vi "MT Display 3DEye.vi"(0 "waveform":T2={"t0"=0.0, "dt"=1.0, "Y"=[]} {"Y" format="%.3f"; "dt" format="%^.2e"; "t0" format="%.4f"}, 1 "3D curve":refnum<k7>, 2 "clear graph":bool, 3 "optional settings":T1={"segment timing (ms)"=100, "occurrence refnum for abort"=refnum}, 5 "symbol rate (Hz)":dbl=1.0 format="%.2f", 7 "eye length (symbol periods)":i32=1, 9 "color":u32(colorbox)=6618880, 11 "error in (no error)":errorcluster, 12 "autoscale":bool, 13 "display size (segments)":i32=100) -> (15 "error out":errorcluster)   [LabVIEW 2020, in "niDMT.lvlib"]
doc: "Divides an input complex-valued waveform into segments and displays those segments as overlapping plots on a 3D graph. The VI determines the segment length based on the <B>symbol rate</B> and <B>eye length</B> parameters."
uses:
  <vilib>/addons/Modulation/niDMT.lvlib
  <vilib>/addons/Modulation/Analog/controls/Complex Data Waveform.ctl
  <vilib>/addons/Modulation/Digital/General/subVIs/mod_Segment Array(complex).vi
  <vilib>/Platform/NI_3dgraph.lvlib
  <vilib>/addons/Modulation/niAMT.lvlib
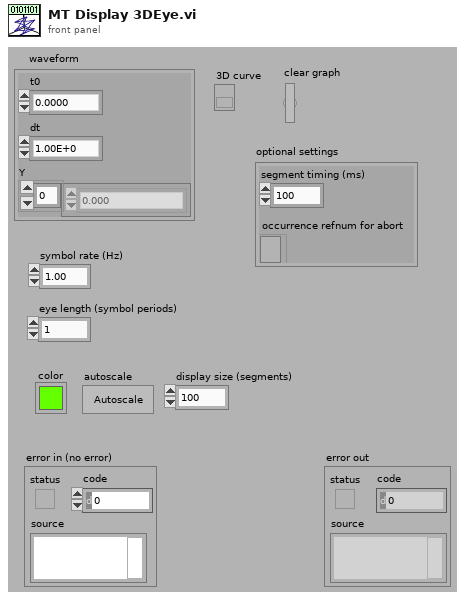
[diagram p1: front panel]
types:
  T1 = cluster{"segment timing (ms)":u32, "occurrence refnum for abort":refnum<k4>}
  T2 = typedef "niAMT.lvlib/Complex Data Waveform.ctl" = cluster{"t0":dbl, "dt":dbl, "Y":cdb[]}
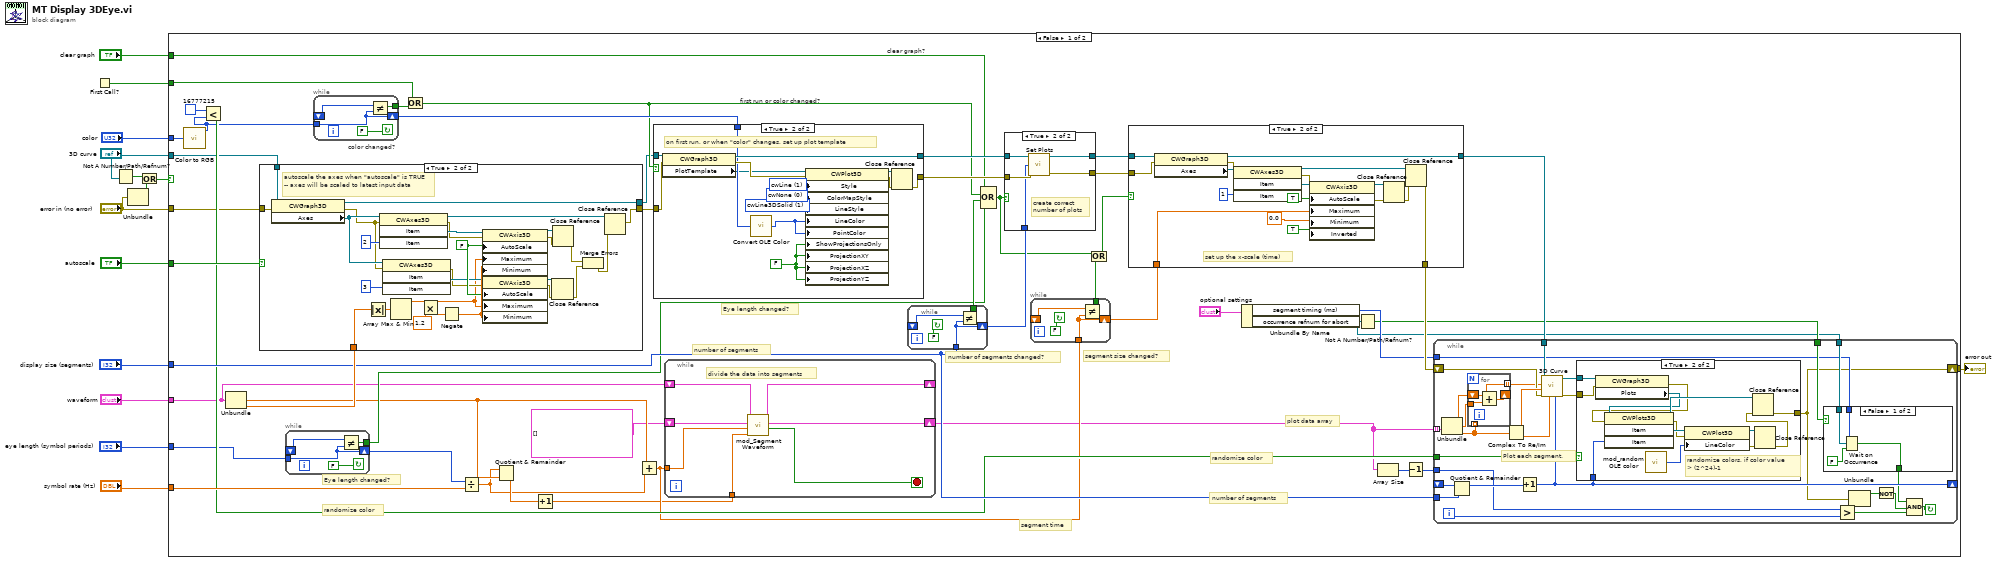
[diagram p0: block diagram]
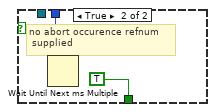
[diagram p2: hidden frame]
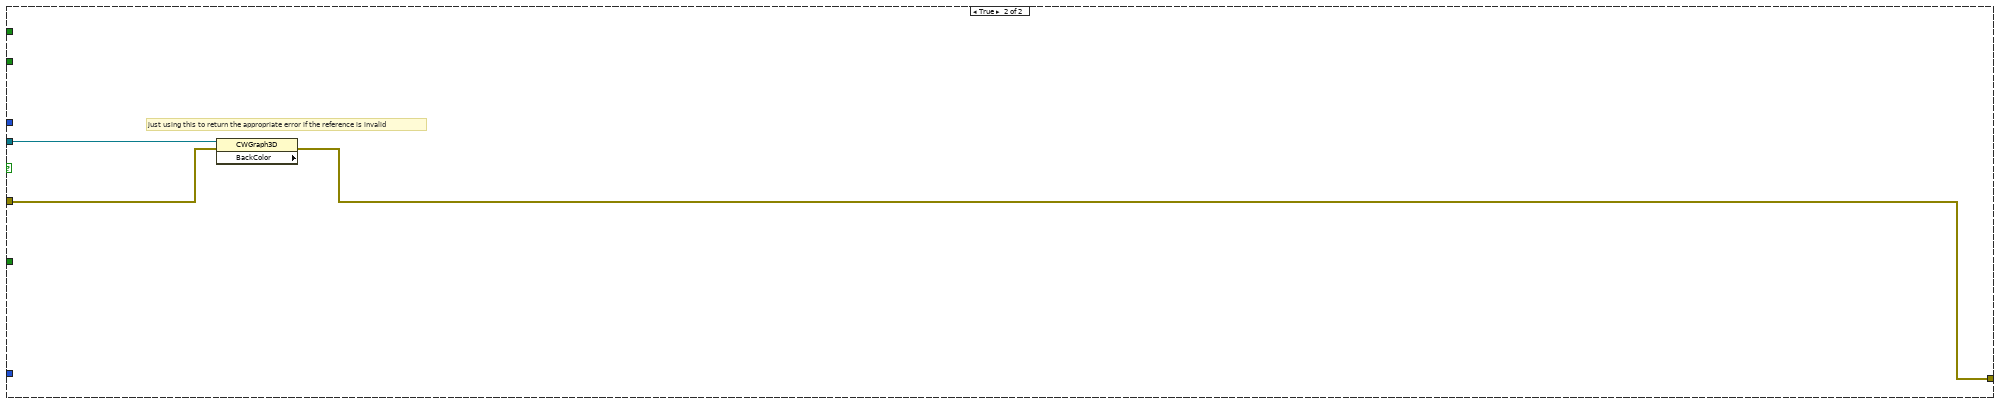
[diagram p8: hidden frame]
diagram:
  n1 = First Call?() -> (First Call?: T/F=w11:bool)
  n2 = Not A Number/Path/Refnum?(number/path/refnum="3D curve") -> (NaN/Path/Refnum?=w2:bool)
  n3 = Unbundle("error in (no error)") -> ("status"=w3:bool)  [unwired: 2 out]
  n4 = Or(x=w2, y=w3) -> (x .or. y?=w1:bool)
  n5 = case shown="False" w1 {
    tunnel: [w59 w206] -> w14
    tunnel: "symbol rate (Hz)" -> [w57 _]
    tunnel: "autoscale" -> [w56 _]
    tunnel: "3D curve" -> [w20 w208]
    tunnel: w11 -> [w51 _]
    tunnel: "display size (segments)" -> [w49 _]
    tunnel: "clear graph" -> [w48 _]
    tunnel: "eye length (symbol periods)" -> [w45 _]
    tunnel: "color" -> [w32 _]
    tunnel: "waveform" -> [w31 _]
    tunnel: "error in (no error)" -> [w26 w207]
    frame False {
      # "plot data array"
      # "number of segments"
      # "randomize color"
      # "segment time"
      # "clear graph?"
      # "first run or color changed?"
      # "Eye length changed?"
      # "number of segments"
      # "randomize color"
      # "segment size changed?"
      # "Eye length changed?"
      # "number of segments changed?"
      # "color changed?"
      n6 = call <vilib>:"Color to RGB.vi"("Color"=w32) -> ("Resolved Color"=w33:u32)  [unwired: 3 out]
      n7 = Less?(x=u32 16777215, y=w33) -> (x < y?=w46:bool)
      n8 = Unbundle(w31) -> ("dt"=w40:dbl, "Y"=w61:cdb[])  [unwired: 1 out]
      n9 = case shown="True" w56 {
        tunnel: w61 -> [_ w198]
        tunnel: w20 -> [w170 w188]
        tunnel: w26 -> [w171 w187]
        tunnel: [w171 w176] -> w27
        tunnel: [w170 w172] -> w19
        frame False {
        }
        frame True {
          w194 = FALSE ("AutoScale")
          # "autoscale the axes when \"autoscale\" is TRUE -- axes will be scaled to latest input data"
          n10 = property class="CWGraph3D"(reference=w188, error in=w187) -> (reference out=w172:refnum<k7>, error out=w185:errorcluster, "Axes"=w186:refnum<k7>)
          n11 = Absolute Value(x=w198) -> (abs(x)=w189:dbl[])
          n12 = invoke class="CWAxes3D" method="Item"(reference=w186, error in=w185, "Item"=2) -> (reference out=w178:refnum<k7>, error out=w184:errorcluster, "Item"=w192:refnum<k7>)  [unwired: 1 in, 1 out]
          n13 = invoke class="CWAxes3D" method="Item"(reference=w186, error in=w185, "Item"=3) -> (error out=w182:errorcluster, "Item"=w193:refnum<k7>)  [unwired: 1 in, 2 out]
          n14 = Array Max & Min(array=w189) -> (max value=w175:dbl)  [unwired: 3 out]
          n15 = Multiply(x=w175, y=1.2) -> (x*y=w174:dbl)
          n16 = Negate(x=w174) -> (-x=w195:dbl)
          n17 = property class="CWAxis3D"(reference=w192, error in=w184, "AutoScale"=w194, "Maximum"=w174, "Minimum"=w195) -> (reference out=w196:refnum<k7>, error out=w183:errorcluster)
          n18 = property class="CWAxis3D"(reference=w193, error in=w182, "AutoScale"=w194, "Maximum"=w174, "Minimum"=w195) -> (reference out=w197:refnum<k7>, error out=w181:errorcluster)
          n19 = Close Reference(reference=w197, error in (no error)=w181) -> (error out=w179:errorcluster)
          n20 = Close Reference(reference=w196, error in (no error)=w183) -> (error out=w180:errorcluster)
          n21 = Merge Errors(w180, w179) -> (w177:errorcluster)
          n22 = Close Reference(reference=w178, error in (no error)=w177) -> (error out=w176:errorcluster)
        }
      }
      n23 = while {
        shift-right: [w137] -> w44
        shift-left: _ -> [w138]
        tunnel: w45 -> [w137]
        tunnel: [w136] -> w43
        stop <- FALSE continue-if-true
        n24 = Not Equal?(x=w138, y=w137) -> (x != y?=w136:bool)
      }
      n25 = while {
        shift-right: [w141] -> w53
        shift-left: _ -> [w142]
        tunnel: w33 -> [w141]
        tunnel: [w140] -> w52
        stop <- FALSE continue-if-true
        n26 = Not Equal?(x=w142, y=w141) -> (x != y?=w140:bool)
      }
      n27 = Or(x=w51, y=w52) -> (x .or. y?=w50:bool)
      n28 = Divide(x=w44, y=w57) -> (x/y=w28:dbl)
      n29 = Quotient & Remainder(x=w28, y=w40) -> (floor(x/y)=w42:dbl)  [unwired: 1 out]
      n30 = Increment(x=w42) -> (x+1=w30:dbl)
      n31 = Add(x=w40, y=w28) -> (x+y=w41:dbl)
      n32 = case shown="True" w50 {
        tunnel: [w143 w145] -> w60
        tunnel: [w144 w158] -> w58
        tunnel: w53 -> [_ w154]
        tunnel: w19 -> [w144 w149]
        tunnel: w27 -> [w143 w148]
        frame False {
        }
        frame True {
          w151 = 1 items=["cwLine"=1, "cwPoint"=2, "cwLinePoint"=3, "cwHiddenLine"=4, "cwSurface"=5, "cwSurfaceLine"=6, "cwSurfaceNormal"=7, "cwContourLine"=8, "cwSurfaceContour"=9] ("Style")
          w152 = 0 items=["cwNone", "cwShaded", "cwColorSpectrum", "cwGrayScale", "cwCustom"] ("ColorMapStyle")
          w153 = 1 items=["cwLine3DNone"=0, "cwLine3DSolid"=1, "cwLine3DDash"=4, "cwLine3DDot"=5, "cwLine3DDashDot"=6] ("LineStyle")
          w157 = FALSE ("ShowProjectionsOnly")
          # "on first run, or when \"color\" changes, set up plot template"
          n33 = property class="CWGraph3D"(reference=w149, error in=w148) -> (reference out=w158:refnum<k7>, error out=w156:errorcluster, "PlotTemplate"=w150:refnum<k7>)
          n34 = call <vilib>:"Convert OLE Color.vi"("color in"=w154) -> ("color out"=w147:u32)
          n35 = property class="CWPlot3D"(reference=w150, error in=w156, "Style"=w151, "ColorMapStyle"=w152, "LineStyle"=w153, "LineColor"=w147, "PointColor"=w147, "ShowProjectionsOnly"=w157, "ProjectionXY"=w157, "ProjectionXZ"=w157, "ProjectionYZ"=w157) -> (reference out=w155:refnum<k7>, error out=w146:errorcluster)
          n36 = Close Reference(reference=w155, error in (no error)=w146) -> (error out=w145:errorcluster)
        }
      }
      n37 = while {
        tunnel: w41 -> [w201]
        shift-right: [w202] -> w24
        shift-left: cluster{dbl, "dt":dbl, cdb[]}[] [] -> [w203]
        shift-right: [w204] -> _
        shift-left: w31 -> [w205]
        tunnel: w30 -> [w200]
        stop <- w199 stop-if-true
        # "divide the data into segments"
        n38 = call-poly <vilib>:"mod_Segment Waveform.vi"("min samples per segment"=w200, "segment time"=w201, "graphs in"=w203, "waveform"=w205) -> ("done?"=w199:bool, "graphs out"=w202:cluster{dbl, "dt":dbl, cdb[]}[], "waveform out"=w204:cluster{"t0":dbl, "dt":dbl, "Y":cdb[]})  [unwired: 5 out]
      }
      n39 = while {
        shift-right: [w168] -> w55
        shift-left: _ -> [w169]
        tunnel: w49 -> [w168]
        tunnel: [w167] -> w54
        stop <- FALSE continue-if-true
        n40 = Not Equal?(x=w169, y=w168) -> (x != y?=w167:bool)
      }
      n41 = Compound Arithmetic op=OR(w48, w50, w54, w43) -> (w34:bool)
      n42 = case shown="True" w34 {
        tunnel: w60 -> [w160 w165]
        tunnel: [w159 w162] -> w39
        tunnel: w58 -> [w159 w164]
        tunnel: [w160 w161] -> w38
        tunnel: w55 -> [_ w163]
        frame False {
        }
        frame True {
          # "create correct number of plots"
          n43 = call <vilib>:"Set Plots.vi"("3D graph"=w164, "# of plots(1)"=w163, "error in (no error)"=w165) -> ("3D graph out"=w162:refnum<k7>, "error out"=w161:errorcluster)  [unwired: 11 out]
        }
      }
      n44 = while {
        shift-right: [w133] -> w37
        shift-left: _ -> [w134]
        tunnel: w41 -> [w133]
        tunnel: [w132] -> w36
        stop <- FALSE continue-if-true
        n45 = Not Equal?(x=w134, y=w133) -> (x != y?=w132:bool)
      }
      n46 = Or(x=w34, y=w36) -> (x .or. y?=w35:bool)
      n47 = case shown="True" w35 {
        tunnel: [w113 w121] -> w22
        tunnel: w39 -> [w113 w118]
        tunnel: w38 -> [w112 w117]
        tunnel: [w112 w116] -> w21
        tunnel: w37 -> [_ w114]
        frame False {
        }
        frame True {
          # "set up the x-scale (time)"
          n48 = property class="CWGraph3D"(reference=w118, error in=w117) -> (reference out=w121:refnum<k7>, error out=w127:errorcluster, "Axes"=w130:refnum<k7>)
          n49 = invoke class="CWAxes3D" method="Item"(reference=w130, error in=w127, "Item"=1) -> (reference out=w122:refnum<k7>, error out=w126:errorcluster, "Item"=w128:refnum<k7>)  [unwired: 1 in, 1 out]
          n50 = property class="CWAxis3D"(reference=w128, error in=w126, "AutoScale"=TRUE, "Maximum"=w114, "Minimum"=0.0, "Inverted"=TRUE) -> (reference out=w124:refnum<k7>, error out=w125:errorcluster)
          n51 = Close Reference(reference=w124, error in (no error)=w125) -> (error out=w123:errorcluster)
          n52 = Close Reference(reference=w122, error in (no error)=w123) -> (error out=w116:errorcluster)
        }
      }
      n53 = Unbundle By Name("optional settings") -> ("segment timing (ms)"=w17:u32, "occurrence refnum for abort"=w15:refnum<k4>)
      n54 = Not A Number/Path/Refnum?(number/path/refnum=w15) -> (NaN/Path/Refnum?=w16:bool)
      n55 = Array Size(array=w24) -> (size(s)=w25:i32)
      n56 = Decrement(x=w25) -> (x-1=w23:i32)
      n57 = while {
        tunnel: w22 -> [w84]
        tunnel: w24 -> [w88] mode=indexing
        shift-right: [w62] -> w59
        shift-left: w21 -> [w85]
        shift-right: [w79] -> _
        shift-left: _ -> [w82]
        tunnel: w49 -> [w83]
        tunnel: w46 -> [w78]
        tunnel: w23 -> [w73]
        tunnel: w17 -> [w63]
        tunnel: w16 -> [w67]
        tunnel: w15 -> [w64]
        i -> [w72]
        stop <- w69 continue-if-true
        # "Plot each segment."
        n58 = Unbundle(w88) -> (w77:dbl, "dt"=w76:dbl, w75:cdb[])
        n59 = Quotient & Remainder(x=w82, y=w83) -> (x-y*floor(x/y)=w81:i32)  [unwired: 1 out]
        n60 = for {
          shift-right: [w95] -> _
          shift-left: w77 -> [w97]
          tunnel: w76 -> [w96]
          tunnel: [w97] -> w74 mode=indexing
          tunnel: w75 -> [_] mode=indexing
          n61 = Add(x=w97, y=w96) -> (x+y=w95:dbl)
        }
        n62 = Complex To Re/Im(x + iy=w75) -> (x=w87:dbl[], y=w86:dbl[])
        n63 = Increment(x=w81) -> (x+1=w79:i32)
        n64 = call <vilib>:"3D Curve.vi"("plot number (1)"=w79, "z vector"=w86, "error in (no error)"=w85, "y vector"=w87, "x vector"=w74, "3D graph"=w84) -> ("error out"=w80:errorcluster, "3D graph out"=w68:refnum<k7>)  [unwired: 4 out]
        n65 = case shown="True" w78 {
          tunnel: w80 -> [w98 w100]
          tunnel: w79 -> [_ w111]
          tunnel: [w98 w103] -> w62
          tunnel: w68 -> [_ w102]
          frame False {
          }
          frame True {
            # "randomize colors, if color value\n> (2^24)-1"
            n66 = property class="CWGraph3D"(reference=w102, error in=w100) -> (error out=w99:errorcluster, "Plots"=w101:refnum<k7>)  [unwired: 1 out]
            n67 = invoke class="CWPlots3D" method="Item"(reference=w101, error in=w99, "Item"=w111) -> (reference out=w110:refnum<k7>, error out=w105:errorcluster, "Item"=w109:refnum<k7>)  [unwired: 1 in, 1 out]
            n68 = call <vilib>:"mod_random OLE color.vi"() -> ("random OLE color"=w106:u32)
            n69 = property class="CWPlot3D"(reference=w109, error in=w105, "LineColor"=w106) -> (reference out=w107:refnum<k7>, error out=w108:errorcluster)
            n70 = Close Reference(reference=w107, error in (no error)=w108) -> (error out=w104:errorcluster)
            n71 = Close Reference(reference=w110, error in (no error)=w104) -> (error out=w103:errorcluster)
          }
        }
        n72 = case shown="False" w67 {
          tunnel: [w90 TRUE] -> w65
          tunnel: w64 -> [w92 _]
          tunnel: w63 -> [w91 w93]
          frame False {
            n73 = Wait on Occurrence(1:FALSE ("ignore previous (T)"), 2:w92, 3:w91) -> (0:w90:bool)
          }
          frame True {
            # "no abort occurence refnum\n supplied"
            n74 = Wait Until Next ms Multiple(millisecond multiple=w93) -> ()  [unwired: 1 out]
          }
        }
        n75 = Greater?(x=w73, y=w72) -> (0:w71:bool)
        n76 = Unbundle(w62) -> ("status"=w70:bool)  [unwired: 2 out]
        n77 = Not(x=w70) -> (.not. x?=w66:bool)
        n78 = Compound Arithmetic op=AND(w65, w66, w71) -> (w69:bool)
      }
    }
    frame True {
      # "just using this to return the appropriate error if the reference is invalid"
      n79 = property class="CWGraph3D" props=["BackColor"](reference=w208, error in=w207) -> (error out=w206:errorcluster)  [unwired: 2 out]
    }
  }
  "error out" <- w14
